vi "SWERVE_DRIVE_ACQUIRE.vi"(6 "Pass_Through_Time":dbl=-1.0 format="%33.4f", 8 "GyroDevRef":T1={"DevStatus"={"status"=FALSE, "code"=0, "source"=""}, "Analog Channel"=enum."AI 1", "Gain (VoltsPerDegree/Second)"=0.0, "Gyro Type"=enum."Analog", "Handle"=0, "SPI Bus"=enum."Invalid", "Device Found"=FALSE, "Sample Rate"=1.0, "Calibrate On Open"=FALSE, "Offset"=0.0} {"Sample Rate" min=0.25 max=100.0 step=0.25}, 9 "in Swerve Module States":T6[](array[typedef]) {"Angle"."SIN" format="%13.4f"; "Angle"."COS" format="%13.4f"; "Angle"."VALUE" format="%13.4f"}, 10 "Swerve IO Reference":T7[](array[typedef]), 11 "in SWERVE_DRIVE_KINEMATICS":T17 {"SavedModuleStates"."Angle"."SIN" format="%13.4f"; "SavedModuleStates"."Angle"."COS" format="%13.4f"; "SavedModuleStates"."Angle"."VALUE" format="%13.4f"; "PrevCoR"."Y" format="%14.3f"; "PrevCoR"."X" format="%14.3f"; "Modules"."Y" format="%14.3f"; "Modules"."X" format="%14.3f"}) -> (0 "out Swerve Module Positions":T4[](array[typedef]) {"Angle"."SIN" format="%13.4f"; "Angle"."COS" format="%13.4f"; "Angle"."VALUE" format="%13.4f"}, 1 "out Swerve Module States":T6[](array[typedef]) {"Angle"."SIN" format="%13.4f"; "Angle"."COS" format="%13.4f"; "Angle"."VALUE" format="%13.4f"}, 2 "Gyro_Heading_Rad":dbl)   [LabVIEW 2019]
uses:
  <vilib>/Rock Robotics/WPI/ThirdParty/JAS_Junk/TrajLib/TypeDef/SWERVE_DRIVE_KINEMATICS.ctl
  <vilib>/Analysis/Matrix/Datatypes/RealMatrix.ctl
  <vilib>/Rock Robotics/WPI/ThirdParty/JAS_Junk/TrajLib/TypeDef/TRANSLATION2D.ctl
  <vilib>/Rock Robotics/WPI/ThirdParty/JAS_Junk/TrajLib/TypeDef/SWERVE_DRIVE_MODULE_STATE.ctl
  <vilib>/Rock Robotics/WPI/ThirdParty/JAS_Junk/TrajLib/TypeDef/ROTATION2D.ctl
  SWERVE_DRIVE_MODULE_TYPDEF.ctl
  <vilib>/Rock Robotics/WPI/MotorControl/WPI_MotorControlDeviceRef.ctl
  <vilib>/Rock Robotics/WPI/MotorControl/WPI_MotorControlType.ctl
  <vilib>/Rock Robotics/SystemInterfaces/DIO/FPGA_DIOPWMChannel.ctl
  <vilib>/Rock Robotics/WPI/PWM/WPI_PWMDeadband.ctl
  <vilib>/Rock Robotics/SystemInterfaces/DIO/FPGA_DIOChannel.ctl
  <vilib>/Rock Robotics/WPI/Encoder/WPI_EncoderDevRef.ctl
  <vilib>/Rock Robotics/SystemInterfaces/Encoder/FPGA_EncoderIdx.ctl
  <vilib>/Rock Robotics/SystemInterfaces/Counter/FPGA_CounterCtrSystemIndex.ctl
  <vilib>/Rock Robotics/WPI/Encoder/WPI_EncoderType.ctl
  <vilib>/Rock Robotics/WPI/ThirdParty/JAS_Junk/TrajLib/TypeDef/SWERVE_DRIVE_MODULE_POSITION.ctl
  <vilib>/Rock Robotics/WPI/Gyro/WPI_GyroDevRef.ctl
  <vilib>/Rock Robotics/SystemInterfaces/AI/FPGA_AIChannel.ctl
  <vilib>/Rock Robotics/SystemInterfaces/spilib/spi_bus.ctl
  <vilib>/Rock Robotics/WPI/ThirdParty/JAS_Junk/TrajLib/VI/Util_GetTime_U32.vi
  <vilib>/Rock Robotics/WPI/ThirdParty/JAS_Junk/TrajLib/MathUtil_InputModulus.vi
  <vilib>/Rock Robotics/WPI/ThirdParty/JAS_Junk/TrajLib/VI/Util_GetTime_U64.vi
  SWERVE_DRIVE_GLOBALS.vi
  <vilib>/Rock Robotics/WPI/ThirdParty/JAS_Junk/TrajLib/Trajectory_Library.lvlib
  <vilib>/Analysis/Matrix/NI_Matrix.lvlib
panel:
  # "Analog"
  # "XRS"
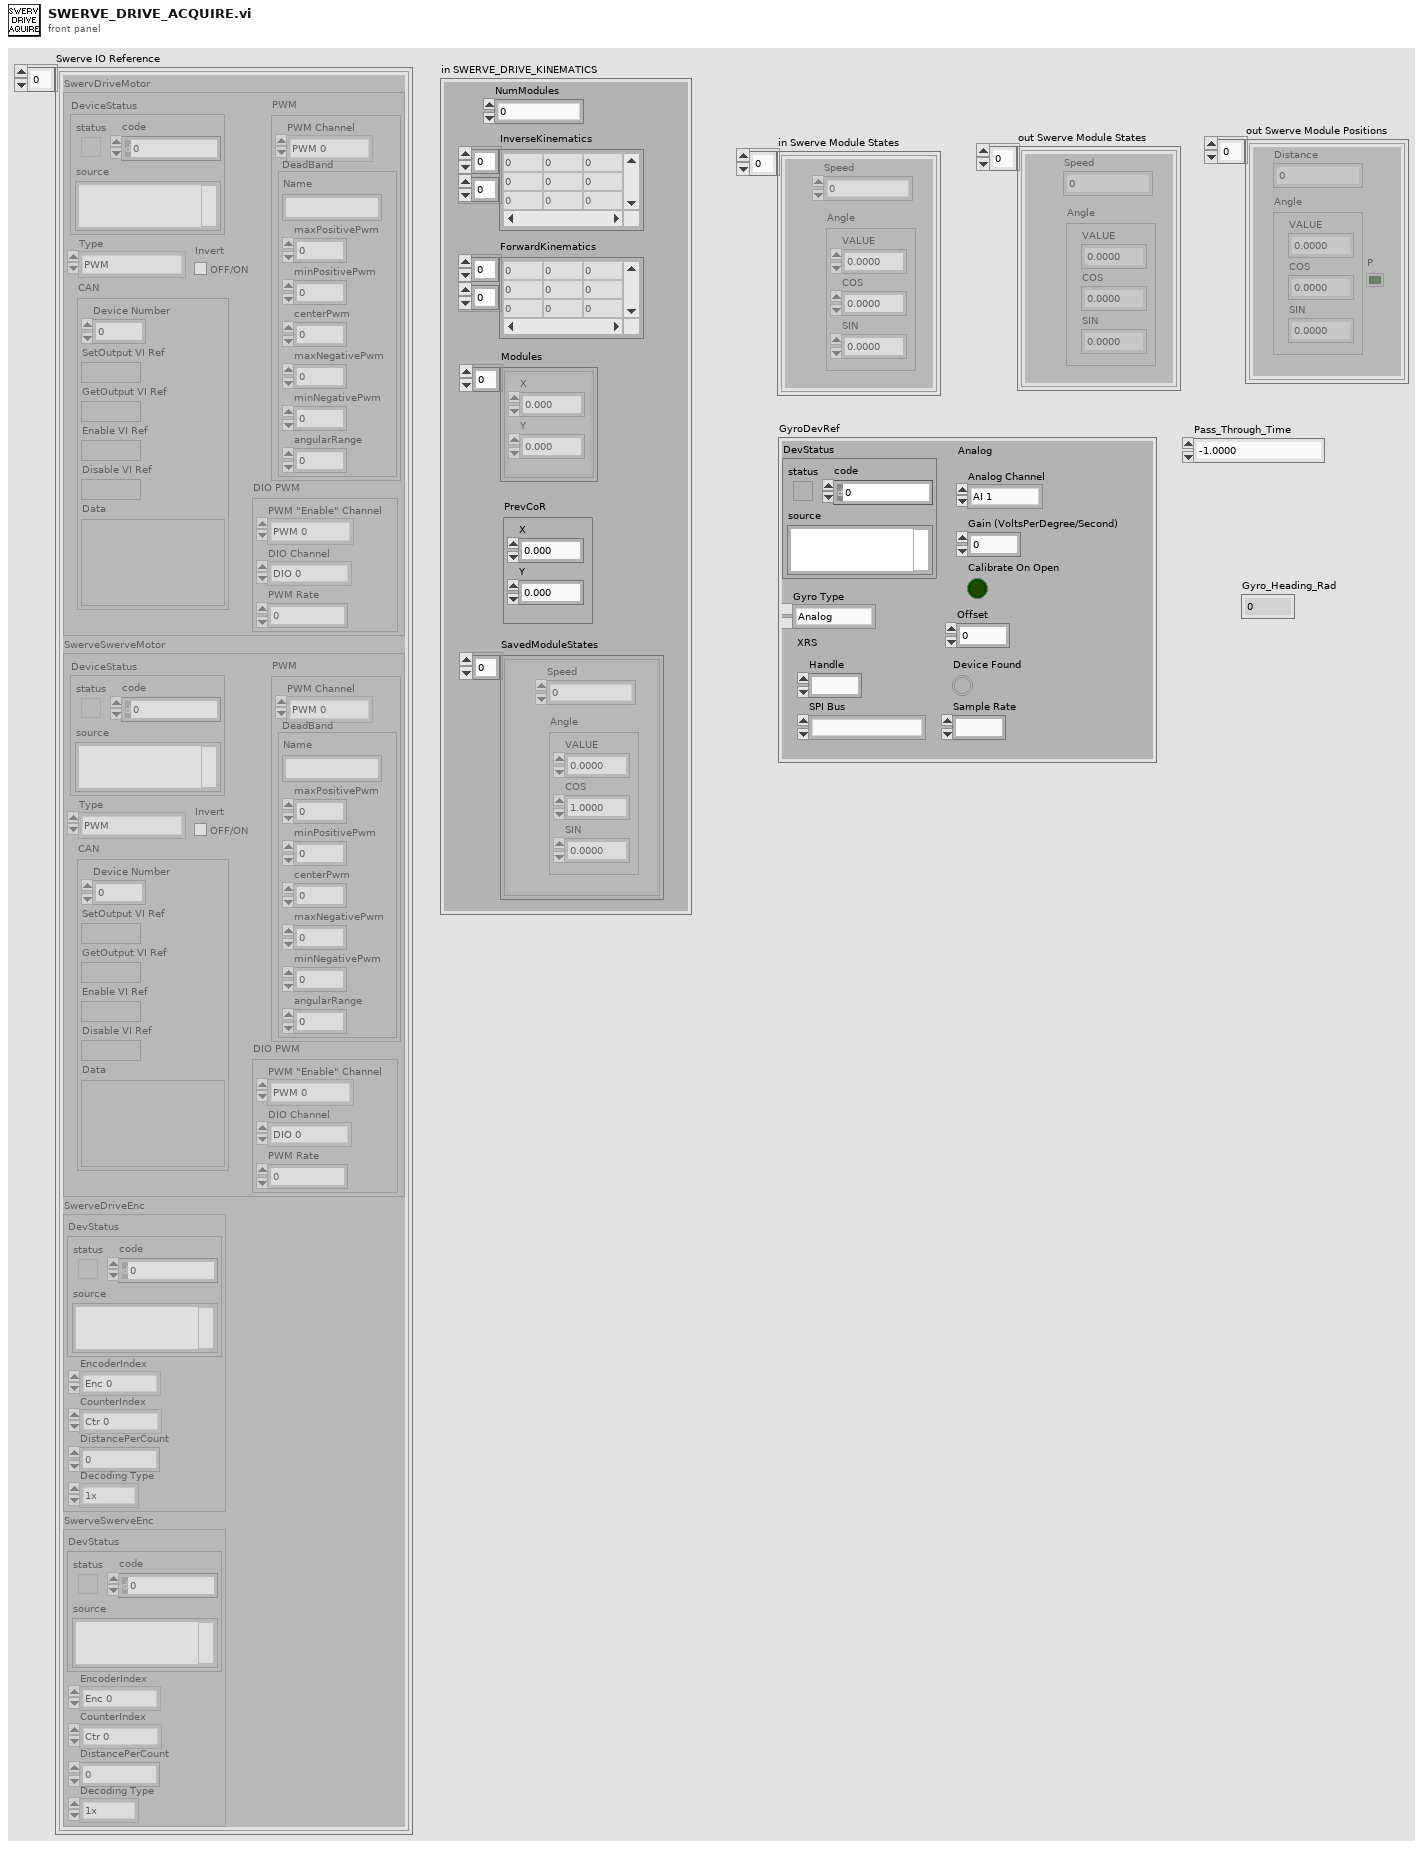
[diagram p1: front panel]
types:
  T1 = typedef "WPI_GyroDevRef.ctl" = cluster{"DevStatus":errorcluster, "Analog Channel":T2, "Gain (VoltsPerDegree/Second)":dbl, "Gyro Type":enum16{"Analog", "XRS450"}, "Handle":i32, "SPI Bus":T3, "Device Found":bool, "Sample Rate":dbl, "Calibrate On Open":bool, "Offset":dbl}
  T2 = typedef "FPGA_AIChannel.ctl" = enum8{"AI 0", "AI 1", "AI 2", "AI 3", "AI MXP 0", "AI MXP 1", "AI MXP 2", "AI MXP 3", "Invalid"}
  T3 = typedef "spi_bus.ctl" = enum16{"SPI On-Board, CS0", "SPI On-Board, CS1", "SPI On-Board, CS2", "SPI On-Board, CS3", "SPI MXP", "Invalid"}
  T4 = typedef "Trajectory_Library.lvlib/SWERVE_DRIVE_MODULE_POSITION.ctl" = cluster{"Distance":dbl, "Angle":T5, "P":bool}
  T5 = typedef "Trajectory_Library.lvlib/ROTATION2D.ctl" = cluster{"VALUE":dbl, "COS":dbl, "SIN":dbl}
  T6 = typedef "Trajectory_Library.lvlib/SWERVE_DRIVE_MODULE_STATE.ctl" = cluster{"Speed":dbl, "Angle":T5}
  T7 = typedef "SWERVE_DRIVE_MODULE_TYPDEF.ctl" = cluster{"SwervDriveMotor":T8, "SwerveSwerveMotor":T8, "SwerveDriveEnc":T13, "SwerveSwerveEnc":T13}
  T8 = typedef "WPI_MotorControlDeviceRef.ctl" = cluster{"DeviceStatus":errorcluster, "Type":T9, "PWM":cluster{"PWM Channel":T10, "DeadBand":T11}, "CAN":cluster{"Device Number":u8, "SetOutput VI Ref":variant, "GetOutput VI Ref":variant, "Enable VI Ref":variant, "Disable VI Ref":variant, "Data":variant}, "Invert":bool, "DIO PWM":cluster{"PWM \"Enable\" Channel":T10, "DIOChannel":T12, "PWM Rate":dbl}}
  T9 = typedef "WPI_MotorControlType.ctl" = enum16{"PWM", "CAN", "DIO PWM"}
  T10 = typedef "FPGA_DIOPWMChannel.ctl" = enum8{"PWM 0", "PWM 1", "PWM 2", "PWM 3", "PWM 4", "PWM 5", "PWM 6", "PWM 7", "PWM 8", "PWM 9", "PWM MXP 0", "PWM MXP 1", "PWM MXP 2", "PWM MXP 3", "PWM MXP 4", "PWM MXP 5", "PWM MXP 6", "PWM MXP 7", "PWM MXP 8", "PWM MXP 9", "Invalid"}
  T11 = typedef "WPI_PWMDeadband.ctl" = cluster{"Name":string, "maxPositivePwm":i32, "minPositivePwm":i32, "centerPwm":i32, "maxNegativePwm":i32, "minNegativePwm":i32, "angularRange":u16}
  T12 = typedef "FPGA_DIOChannel.ctl" = enum8{"DIO 0", "DIO 1", "DIO 2", "DIO 3", "DIO 4", "DIO 5", "DIO 6", "DIO 7", "DIO 8", "DIO 9", "DIO MXP 0", "DIO MXP 1", "DIO MXP 2", "DIO MXP 3", "DIO MXP 4", "DIO MXP 5", "DIO MXP 6", "DIO MXP 7", "DIO MXP 8", "DIO MXP 9", "DIO MXP 10", "DIO MXP 11", "DIO MXP 12", "DIO MXP 13", "DIO MXP 14", "DIO MXP 15", "SPI Port CS1", "SPI Port CS2", "SPI Port CS3", "SPI Port MISO", "SPI Port MOSI", "Invalid"}
  T13 = typedef "WPI_EncoderDevRef.ctl" = cluster{"DevStatus":errorcluster, "EncoderIndex":T14, "CounterIndex":T15, "DistancePerCount":dbl, "Decoding Type":T16}
  T14 = typedef "FPGA_EncoderIdx.ctl" = enum8{"Enc 0", "Enc 1", "Enc 2", "Enc 3", "Enc 4", "Enc 5", "Enc 6", "Enc 7", "Invalid"}
  T15 = typedef "FPGA_CounterCtrSystemIndex.ctl" = enum8{"Ctr 0", "Ctr 1", "Ctr 2", "Ctr 3", "Ctr 4", "Ctr 5", "Ctr 6", "Ctr 7", "Invalid"}
  T16 = typedef "WPI_EncoderType.ctl" = enum16{"1x", "2x", "4x"}
  T17 = typedef "Trajectory_Library.lvlib/SWERVE_DRIVE_KINEMATICS.ctl" = cluster{"NumModules":i32, "InverseKinematics":T18, "ForwardKinematics":T18, "Modules":T19[], "PrevCoR":T19, "SavedModuleStates":T6[]}
  T18 = typedef "NI_Matrix.lvlib/RealMatrix.ctl" = dbl[][]
  T19 = typedef "Trajectory_Library.lvlib/TRANSLATION2D.ctl" = cluster{"X":dbl, "Y":dbl}
  T20 = typedef "Trajectory_Library.lvlib/CHASSIS_SPEEDS.ctl" = cluster{"vX":dbl, "vY":dbl, "vOmega":dbl}
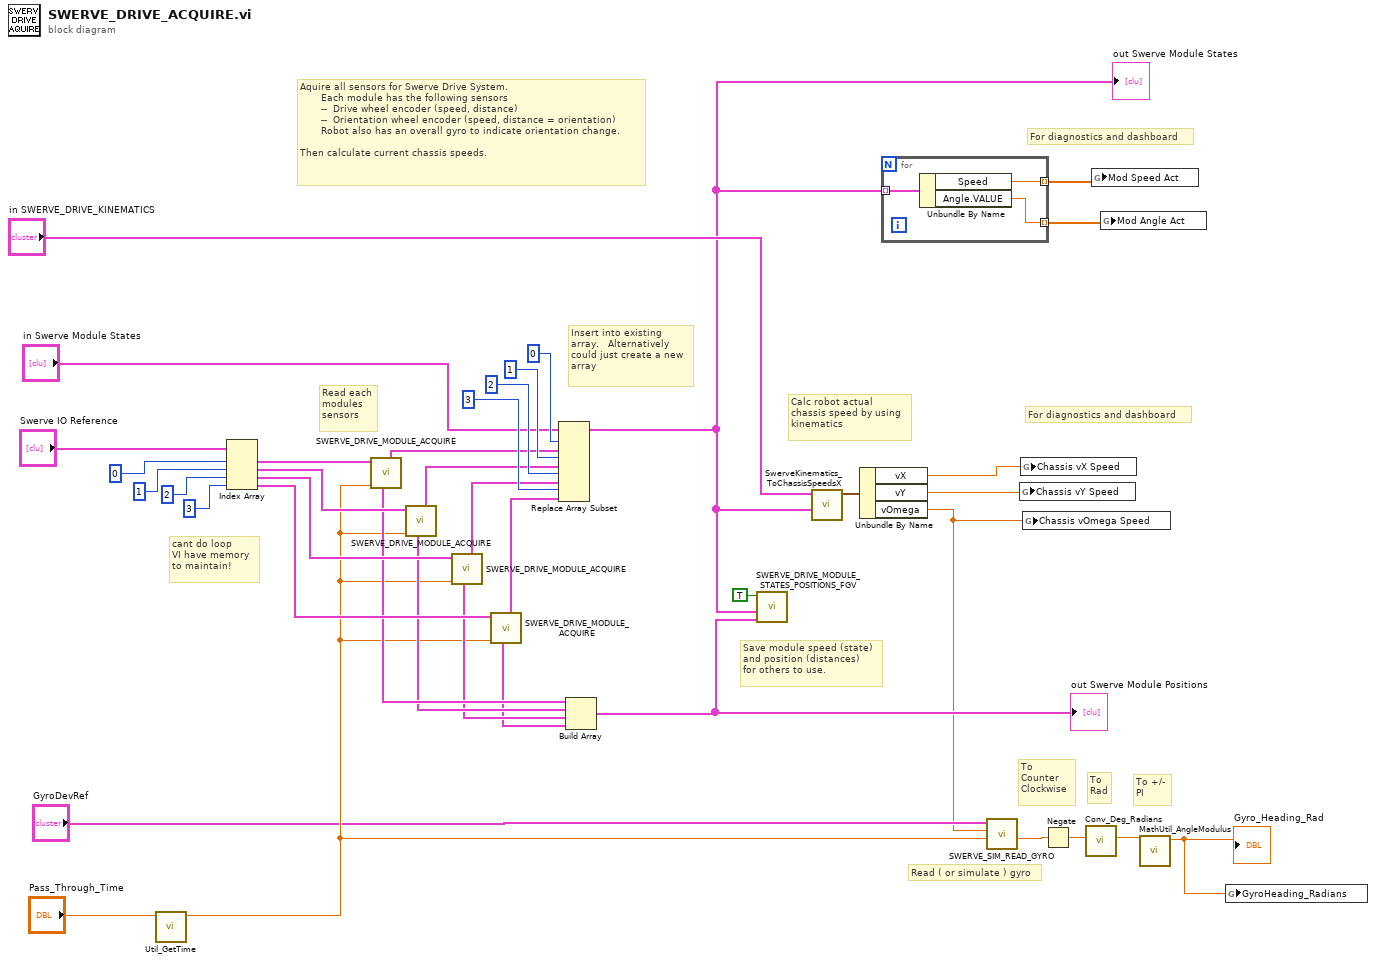
[diagram p0: block diagram]
diagram:
  # "For diagnostics and dashboard"
  # "For diagnostics and dashboard"
  # "Read each\nmodules\nsensors"
  # "To\nCounter\nClockwise"
  # "To +/-\nPI"
  # "To\nRad"
  # "Read ( or simulate ) gyro"
  # "Aquire all sensors for Swerve Drive System.\n       Each module has the following sensors\n       --  Drive wheel encoder (speed, distance)\n       --  Orientation wheel encoder (speed, distance = orientation)\n       Robot also has an overall gyro to indicate orientation change.\n\nThen calculate current chassis speeds."
  # "Insert into existing\narray.   Alternatively\ncould just create a new\narray"
  # "Calc robot actual\nchassis speed by using\nkinematics"
  # "Save module speed (state)\nand position (distances)\nfor others to use."
  # "cant do loop\nVI have memory\nto maintain!"
  n1 = call <vilib>:"Util_GetTime.vi"("Pass_Through_Time"="Pass_Through_Time") -> ("FPGA_Time_Seconds"=w9:dbl)  [unwired: 8 in, 2 out]
  n2 = Index Array(array="Swerve IO Reference", index #1=0 ("index"), index #2=1 ("index"), index #3=2 ("index"), index #4=3 ("index")) -> (element #1=w24:T7, element #2=w25:T7, element #3=w26:T7, element #4=w32:T7)
  n3 = call "SWERVE_DRIVE_MODULE_ACQUIRE.vi"("Pass_Through_Time"=w9, "Swerve Module TypDef"=w24) -> ("Swerve Module State"=w20:T6, "SWERVE DRIVE MODULE POSITION"=w18:T4)  [unwired: 3 in, 5 out]
  n4 = call "SWERVE_DRIVE_MODULE_ACQUIRE.vi"("Pass_Through_Time"=w9, "Swerve Module TypDef"=w25) -> ("Swerve Module State"=w23:T6, "SWERVE DRIVE MODULE POSITION"=w17:T4)  [unwired: 3 in, 5 out]
  n5 = call "SWERVE_DRIVE_MODULE_ACQUIRE.vi"("Pass_Through_Time"=w9, "Swerve Module TypDef"=w26) -> ("Swerve Module State"=w22:T6, "SWERVE DRIVE MODULE POSITION"=w16:T4)  [unwired: 3 in, 5 out]
  n6 = call "SWERVE_DRIVE_MODULE_ACQUIRE.vi"("Pass_Through_Time"=w9, "Swerve Module TypDef"=w32) -> ("Swerve Module State"=w33:T6, "SWERVE DRIVE MODULE POSITION"=w15:T4)  [unwired: 3 in, 5 out]
  n7 = Replace Array Subset(array="in Swerve Module States", new element #1=w20, index #1=0 ("index"), new element #2=w23, index #2=1 ("index"), new element #3=w22, index #3=2 ("index"), new element #4=w33, index #4=3 ("index")) -> (w12:T6[])
  "out Swerve Module States" <- w12
  n8 = Build Array(w18, w17, w16, w15) -> (w14:T4[])
  "out Swerve Module Positions" <- w14
  n9 = call "SWERVE_DRIVE_MODULE_STATES_POSITIONS_FGV.vi"("in Current Module Positions"=w14, "in Current Module States"=w12, "WRITE"=TRUE) -> ()  [unwired: 7 in, 2 out]
  n10 = call <vilib>:"SwerveKinematics_ToChassisSpeedsX.vi"("WheelStates"=w12, "in SWERVE_DRIVE_KINEMATICS"="in SWERVE_DRIVE_KINEMATICS") -> ("Chassis Speed"=w39:T20)  [unwired: 9 in]
  n11 = Unbundle By Name(w39) -> ("vX"=w5:dbl, "vY"=w6:dbl, "vOmega"=w7:dbl)
  n12 = for {
    tunnel: w12 -> [w42] mode=indexing
    tunnel: [w41] -> w10 mode=indexing
    tunnel: [w40] -> w11 mode=indexing
    n13 = Unbundle By Name(w42) -> ("Speed"=w40:dbl, "Angle.VALUE"=w41:dbl)
  }
  n14 = call "SWERVE_SIM_READ_GYRO.vi"("FPGA_Time_Seconds"=w9, "vOmega"=w7, "GyroDevRef"="GyroDevRef") -> ("Gyro_Cont_Deg"=w4:dbl)  [unwired: 8 in]
  n15 = global write "SWERVE_DRIVE_GLOBALS.vi" "Chassis vY Speed"(w6) -> ()
  n16 = global write "SWERVE_DRIVE_GLOBALS.vi" "Chassis vX Speed"(w5) -> ()
  n17 = global write "SWERVE_DRIVE_GLOBALS.vi" "Chassis vOmega Speed"(w7) -> ()
  n18 = Negate(x=w4) -> (-x=w3:dbl)
  n19 = call <vilib>:"Conv_Deg_Radians.vi"("Degress"=w3) -> ("Radians"=w2:dbl)  [unwired: 10 in]
  n20 = global write "SWERVE_DRIVE_GLOBALS.vi" "Mod Speed Act"(w11) -> ()
  n21 = global write "SWERVE_DRIVE_GLOBALS.vi" "Mod Angle Act"(w10) -> ()
  n22 = call <vilib>:"MathUtil_AngleModulus.vi"("InputAngle"=w2) -> ("ModulsAngle"=w1:dbl)  [unwired: 10 in]
  "Gyro_Heading_Rad" <- w1
  n23 = global write "SWERVE_DRIVE_GLOBALS.vi" "GyroHeading_Radians"(w1) -> ()
